vi "Run View.vi"(8 "error in (no error)":errorcluster, 11 "base view in":refnum<class "base view.lvclass">) -> (0 "error out":errorcluster, 3 "base view out":refnum<class "base view.lvclass">)   [LabVIEW 2022 SP3, in "base view.lvclass"]
uses:
  base view.lvclass
  View.vi
  Accessors/Write View Refnum.vi
  base view.lvclass/base view.ctl
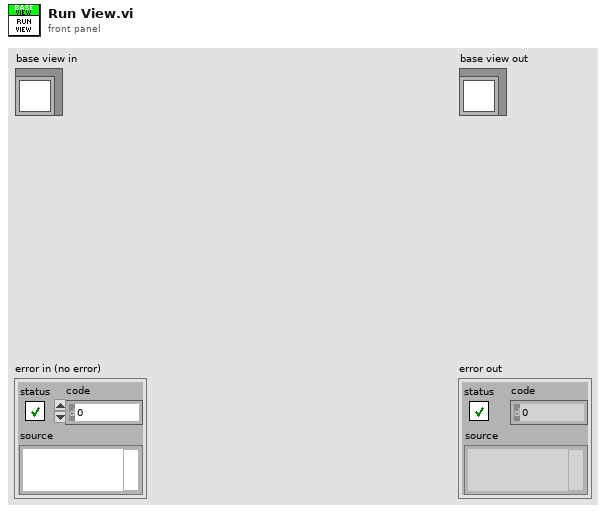
[diagram p1: front panel]
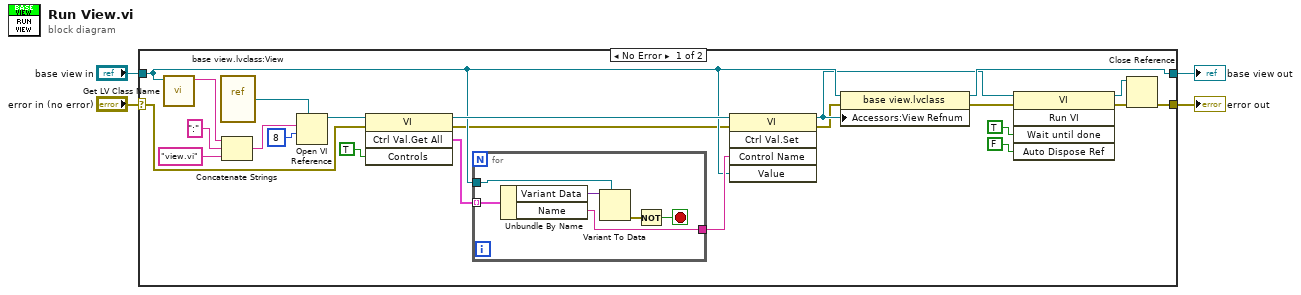
[diagram p0: block diagram]
diagram:
  n1 = case shown="No Error" "error in (no error)" {
    selector: "error in (no error)" -> [w9 w35]
    tunnel: [w5 w35] -> w3
    tunnel: [w15 w34] -> w1
    tunnel: "base view in" -> [w16 w34]
    frame No Error {
      n2 = call <vilib>:"Get LV Class Name.vi"("object"=w16) -> ("class name"=w27:string)  [unwired: 9 in, 1 out]
      n3 = vi-ref "base view.lvclass:View.vi"() -> (w22:refnum<vi>)
      n4 = Concatenate Strings(w27, ":", "view.vi" ("string")) -> (w24:string)
      n5 = Open VI Reference(type specifier VI Refnum (for type only)=w22, vi path=w24, options=8) -> (vi reference=w21:refnum<vi>)  [unwired: 3 in, 1 out]
      n6 = invoke class="VI" method="Ctrl Val.Get All"(reference=w21, error in=w9, "Controls"=TRUE) -> (reference out=w18:refnum<vi>, error out=w8:errorcluster, "Get All Control Values Variant"=w19:cluster{"Name":string, "Variant Data":variant}[])  [unwired: 1 in, 1 out]
      n7 = for {
        tunnel: w19 -> [w33] mode=indexing
        tunnel: w16 -> [w31]
        tunnel: [w30] -> w17
        stop <- w28 stop-if-true
        n8 = Unbundle By Name(w33) -> ("Variant Data"=w32:variant, "Name"=w30:string)
        n9 = Variant To Data(type=w31, Variant=w32) -> (error out=w29:errorcluster)  [unwired: 1 in, 1 out]
        n10 = Not(x=w29) -> (.not. x?=w28:bool)
      }
      n11 = invoke class="VI" method="Ctrl Val.Set"(reference=w18, error in=w8, "Control Name"=w17, "Value"=w16) -> (reference out=w14:refnum<vi>, error out=w7:errorcluster)  [unwired: 1 in, 3 out]
      n12 = property class="base view.lvclass"(reference=w16, error in=w7, "Accessors:View Refnum"=w14) -> (reference out=w15:refnum<class "base view.lvclass">, error out=w6:errorcluster)
      n13 = invoke class="VI" method="Run VI"(reference=w14, error in=w6, "Wait until done"=TRUE ("Wait Until Done"), "Auto Dispose Ref"=FALSE ("Auto Dispose Reference")) -> (reference out=w10:refnum<vi>, error out=w11:errorcluster)  [unwired: 1 in, 3 out]
      n14 = Close Reference(reference=w10, error in (no error)=w11) -> (error out=w5:errorcluster)
    }
    frame Error {
    }
  }
  "error out" <- w3
  "base view out" <- w1
